vi "Configure Current Output.vi"(7 "Triggered Current (0 A)":dbl, 8 "error in (no error)":errorcluster, 9 "Immediate Current (0 A)":dbl, 10 "Transient Operation (0: Fixed)":i32(ring) items=["Fixed", "Step"], 11 "VISA resource name":refnum<visa-resource-name>) -> (0 "error out":errorcluster, 3 "VISA resource name out":refnum<visa-resource-name>)   [LabVIEW 2017, in "Keysight N8900 Series.lvlib"]
doc: "Configures the current transient mode and output current level."
uses:
  Keysight N8900 Series.lvlib
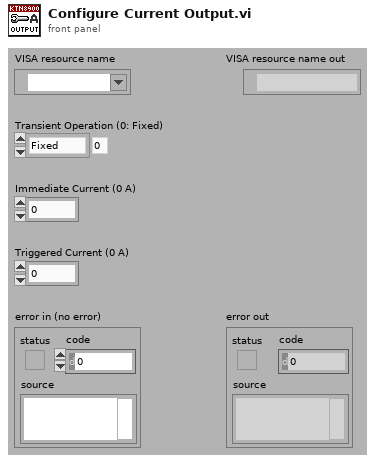
[diagram p1: front panel]
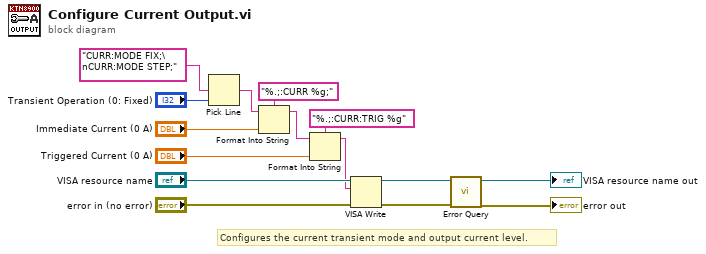
[diagram p0: block diagram]
diagram:
  # "Configures the current transient mode and output current level."
  n1 = Pick Line(multi-line string="CURR:MODE FIX;\nCURR:MODE STEP;", line index="Transient Operation (0: Fixed)") -> (output string=w5:string)  [unwired: 1 in]
  n2 = Format Into String(format string="%.;:CURR %g;", initial string=w5, "Immediate Current (0 A)") -> (resulting string=w2:string)  [unwired: 1 in, 1 out]
  n3 = Format Into String(format string="%.;:CURR:TRIG %g", initial string=w2, "Triggered Current (0 A)") -> (resulting string=w1:string)  [unwired: 1 in, 1 out]
  n4 = VISA Write(VISA resource name="VISA resource name", write buffer=w1, error in (no error)="error in (no error)") -> (VISA resource name out=w11:refnum<visa-resource-name>, error out=w10:errorcluster)  [unwired: 1 out]
  n5 = call "Error Query.vi"("error in (no error)"=w10, "VISA resource name"=w11) -> ("error out"=→"error out":errorcluster, "VISA resource name out"=→"VISA resource name out":refnum<visa-resource-name>)  [unwired: 6 in, 2 out]
